vi "UDP Rx Process.vi"(10 "Parameters":variant, 11 "Process":refnum<class "Process.lvclass">) -> ()   [LabVIEW 2016, in "UDP-Custom-Device Engine.lvlib"]
uses:
  UDP-Custom-Device Engine.lvlib
  <vilib>/NI/NIVS Inline Async API/_VS Inline Async API/Process/Process.lvclass
  <vilib>/NI/NIVS Inline Async API/_VS Inline Async API/Process/Process.lvclass/Process.ctl
  <vilib>/NI Veristand/VeriStand Data/Library/Byte Buffer/Byte Buffer.lvclass/Byte Buffer.ctl
  <vilib>/NI/NIVS Inline Async API/_Data Access Engine/Access Type Classes/Write/Write.lvclass/Write.ctl
  <vilib>/NI/NIVS Inline Async API/_Data Access Engine/Data Access Engine/Methods/Write.Data.vi
  <vilib>/NI/NIVS Inline Async API/_VS Inline Async API/Process/Data Member Access/Read Data Access.vi
  <vilib>/NI/NIVS Inline Async API/_VS Inline Async API/Error Handling Process/SubVIs/Error.ConvertArray.vi
  <vilib>/NI Veristand/VeriStand Data/Library/Byte Buffer/Byte Buffer.Mapping.Read.vi
  <vilib>/NI Veristand/VeriStand Data/Library/Pointer Operations/Pointer.Read.vi
  <vilib>/NI Veristand/VeriStand Data/Library/Pointer Operations/Pointer.Read (DBL).vi
  <vilib>/NI/NIVS Inline Async API/_Data Access Engine/Access Type Classes/Write/Write.ProcessData.vi
  <vilib>/NI Veristand/VeriStand Data/Library/Type Conversion/Type Conversion.To Double.vi
  <vilib>/NI Veristand/VeriStand Data/Library/Type Conversion/Type Conversion.To Double (U16).vi
  <vilib>/NI Veristand/VeriStand Data/Library/Byte Buffer/Byte Buffer.Read.Typed Array.vi
  <vilib>/NI Veristand/VeriStand Data/Library/Memory Management/Memory Management.MoveDblBlock.Read (Double).vi
  <vilib>/NI Veristand/VeriStand Data/Library/Utilities/Utilities.Buffer.Double.vi
  <vilib>/NI Veristand/VeriStand Data/Library/Pointer Operations/Pointer.In-Place Read (DBL).vi
  <vilib>/NI Veristand/VeriStand Data/Library/Utilities/Utilities.Sizeof.Array.vi
  <vilib>/NI Veristand/VeriStand Data/Library/Byte Buffer/Byte Buffer.Read.vi
  <vilib>/NI Veristand/VeriStand Data/Library/Byte Buffer/Byte Buffer.Read (1D Boolean).vi
  <vilib>/NI Veristand/VeriStand Data/Library/Type Conversion/Type Conversion.To Double.Subset.vi
  <vilib>/NI Veristand/VeriStand Data/Library/Type Conversion/Type Conversion.To Double.Subset (1D Boolean).vi
  <vilib>/NI Veristand/VeriStand Data/Library/Byte Buffer/Byte Buffer.Read (1D SGL).vi
  <vilib>/NI Veristand/VeriStand Data/Library/Type Conversion/Type Conversion.To Double.Subset (1D SGL).vi
  <vilib>/NI Veristand/VeriStand Data/Library/Byte Buffer/Byte Buffer.Read (1D DBL).vi
  <vilib>/NI Veristand/VeriStand Data/Library/Byte Buffer/Byte Buffer.Read (1D I8).vi
  <vilib>/NI Veristand/VeriStand Data/Library/Type Conversion/Type Conversion.To Double.Subset (1D I8).vi
  <vilib>/NI Veristand/VeriStand Data/Library/Byte Buffer/Byte Buffer.Read (1D I16).vi
  <vilib>/NI Veristand/VeriStand Data/Library/Type Conversion/Type Conversion.To Double.Subset (1D I16).vi
  <vilib>/NI Veristand/VeriStand Data/Library/Byte Buffer/Byte Buffer.Read (1D I32).vi
  <vilib>/NI Veristand/VeriStand Data/Library/Type Conversion/Type Conversion.To Double.Subset (1D I32).vi
  <vilib>/NI Veristand/VeriStand Data/Library/Byte Buffer/Byte Buffer.Read (1D I64).vi
  <vilib>/NI Veristand/VeriStand Data/Library/Type Conversion/Type Conversion.To Double.Subset (1D I64).vi
  <vilib>/NI Veristand/VeriStand Data/Library/Byte Buffer/Byte Buffer.Read (1D U8).vi
  <vilib>/NI Veristand/VeriStand Data/Library/Type Conversion/Type Conversion.To Double.Subset (1D U8).vi
  <vilib>/NI Veristand/VeriStand Data/Library/Byte Buffer/Byte Buffer.Read (1D U16).vi
  <vilib>/NI Veristand/VeriStand Data/Library/Type Conversion/Type Conversion.To Double.Subset (1D U16).vi
  <vilib>/NI Veristand/VeriStand Data/Library/Byte Buffer/Byte Buffer.Read (1D U32).vi
  <vilib>/NI Veristand/VeriStand Data/Library/Type Conversion/Type Conversion.To Double.Subset (1D U32).vi
  <vilib>/NI Veristand/VeriStand Data/Library/Byte Buffer/Byte Buffer.Read (1D U64).vi
  <vilib>/NI Veristand/VeriStand Data/Library/Type Conversion/Type Conversion.To Double.Subset (1D U64).vi
  <vilib>/NI Veristand/VeriStand Data/Library/Utilities/Utilities.Sizeof.Scalar.vi
  <vilib>/NI Veristand/VeriStand Data/Library/Type Conversion/Type Conversion.To Double (1D Boolean).vi
  <vilib>/NI Veristand/VeriStand Data/Library/Type Conversion/Type Conversion.To Double (1D SGL).vi
  <vilib>/NI Veristand/VeriStand Data/Library/Type Conversion/Type Conversion.To Double (1D I8).vi
  <vilib>/NI Veristand/VeriStand Data/Library/Type Conversion/Type Conversion.To Double (1D I16).vi
  <vilib>/NI Veristand/VeriStand Data/Library/Type Conversion/Type Conversion.To Double (1D I32).vi
  <vilib>/NI Veristand/VeriStand Data/Library/Type Conversion/Type Conversion.To Double (1D I64).vi
  <vilib>/NI Veristand/VeriStand Data/Library/Type Conversion/Type Conversion.To Double (1D U8).vi
  <vilib>/NI Veristand/VeriStand Data/Library/Type Conversion/Type Conversion.To Double (1D U16).vi
  <vilib>/NI Veristand/VeriStand Data/Library/Type Conversion/Type Conversion.To Double (1D U32).vi
  <vilib>/NI Veristand/VeriStand Data/Library/Type Conversion/Type Conversion.To Double (1D U64).vi
  <vilib>/NI Veristand/VeriStand Data/Library/Byte Buffer/Byte Buffer.Set Buffer.vi
  <vilib>/NI Veristand/VeriStand Data/Library/Memory Management/Memory Management.Handle Return.vi
  <vilib>/NI/NIVS Inline Async API/_Data Access Engine/Data Access Engine/Data Access Engine.lvclass
  <vilib>/NI Veristand/VeriStand Data/Library/VeriStand Data.lvlib
panel:
  out "length":i32
  out "Rx Packet":string
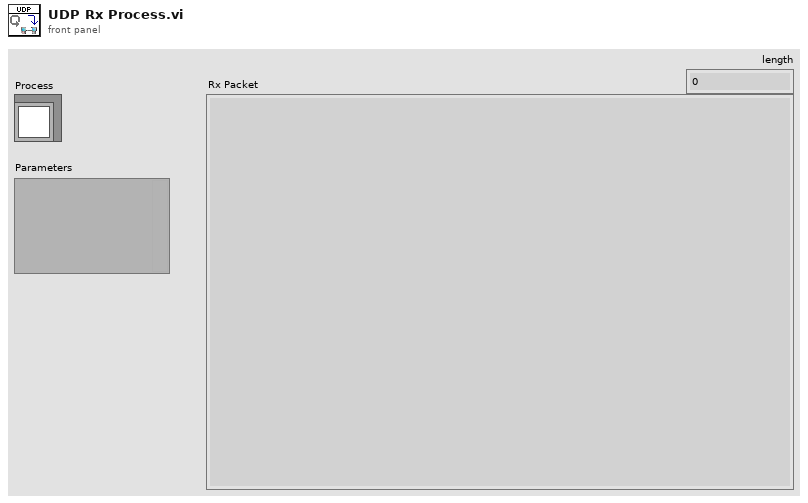
[diagram p1: front panel]
types:
  T1 = typedef "UDP-Custom-Device Engine.lvlib/Engine - Rx Loop Data.ctl" = cluster{"General Resources":T2, "Header Details":T4, "Data Conversion":T5, "Runtime Resources":T7, "New Data Support":T8, "Channel Resources":T10, "Debug Resources":T12}
  T2 = typedef "UDP-Custom-Device Engine.lvlib/Engine - General Resources.ctl" = cluster{"Packet Name":string, "Packet ID":i32, "Local IP Address":string, "Local Port":i32, "Multicast":bool, "Multicast IP Address":u32, "Header Info":bool[], "Byte Order":enum16{"big-endian, network order", "native, host order", "little-endian"}, "Channel Data Types":T3[], "Duplex Packets":refnum<data-value>}
  T3 = typedef "VeriStand Data.lvlib/Typedefs.Data Types.ctl" = enum16{"Boolean", "Single", "Double", "I8", "I16", "I32", "I64", "U8", "U16", "U32", "U64"}
  T4 = typedef "UDP-Custom-Device Shared.lvlib/Shared - Header Details.ctl" = cluster{"Packet Size":u16, "Protocol Revision":u8, "System Definition Version":u64, "Source Node Name":string, "Packet ID":u32, "Number of Channels":u32, "Static Header Size":u16, "Total Header Size":u16}
  T5 = typedef "UDP-Custom-Device Engine.lvlib/Engine - Data Conversion Config.ctl" = cluster{"Byte Buffer":refnum<class "Byte Buffer.lvclass">, "Data Pointers":u64[], "Channel Count":i32, "Mappings":T6[], "Static Header Payload":string, "Packet Count":dbl, "Packet Size":i32}
  T6 = typedef "VeriStand Data.lvlib/Byte Buffer.lvclass/Byte Buffer.Mapping.ctl" = cluster{"pointer":u64, "count":i32, "buffer offset":i32, "data type":T3}
  T7 = typedef "UDP-Custom-Device Engine.lvlib/Engine - Rx Runtime Resources.ctl" = cluster{"Connection ID":refnum<k16>, "Timeout":i32}
  T8 = typedef "UDP-Custom-Device Engine.lvlib/Engine - Rx New Data Options Support.ctl" = cluster{"New Data Option":T9, "Packet Count":dbl}
  T9 = typedef "UDP-Custom-Device Shared.lvlib/Shared - New Data Options.ctl" = enum16{"Timeout Reset", "Counter"}
  T10 = typedef "UDP-Custom-Device Engine.lvlib/Engine - Rx Channel Refs.ctl" = cluster{"Receive Channels":T11, "New Data":T11, "Port":T11}
  T11 = typedef "Data Access Engine.lvlib/Data Access Engine.lvclass/Write.DVR.ctl" = refnum<data-value>
  T12 = typedef "UDP-Custom-Device Engine.lvlib/Engine - Debug Resources.ctl" = cluster{"Debug Mode":bool, "Debug Log File":refnum<file>, "Packet Name":string}
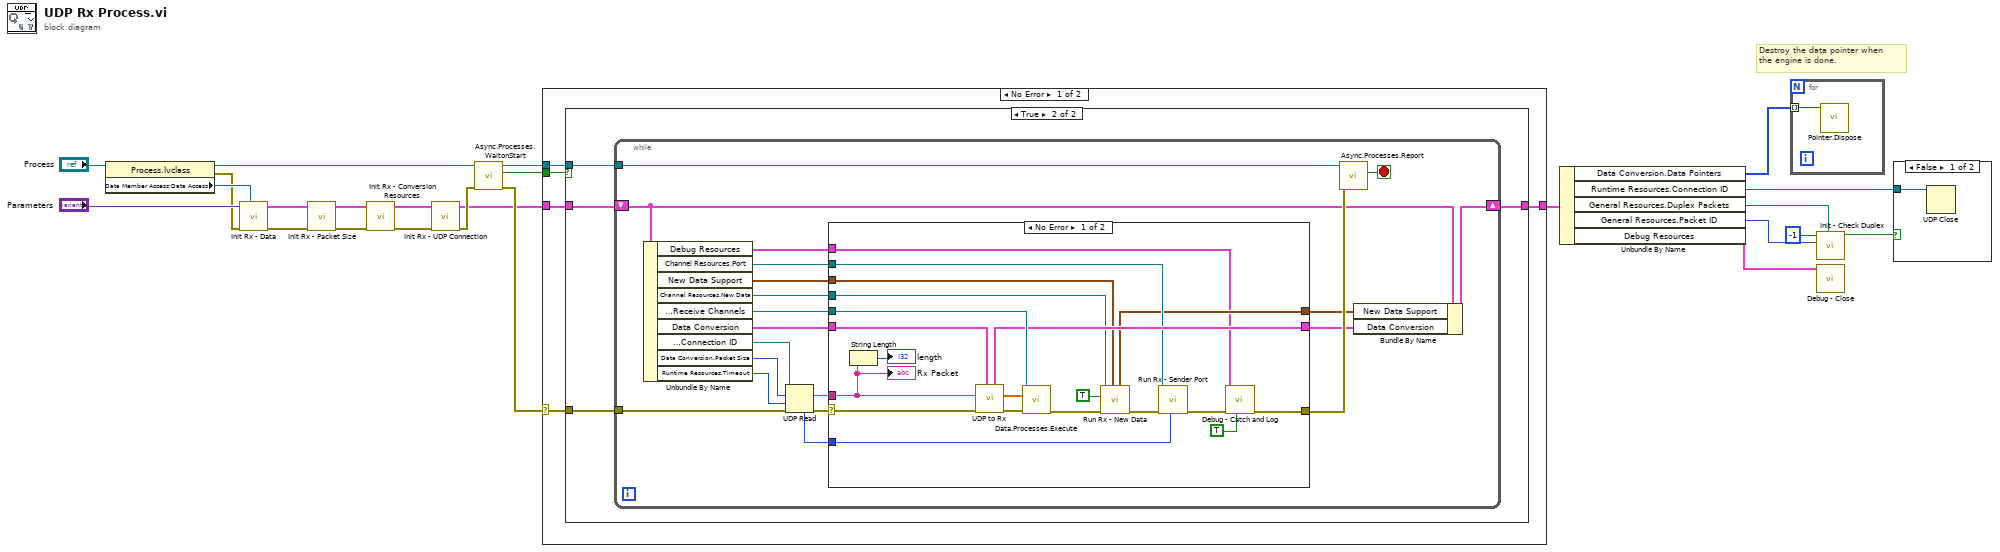
[diagram p0: block diagram]
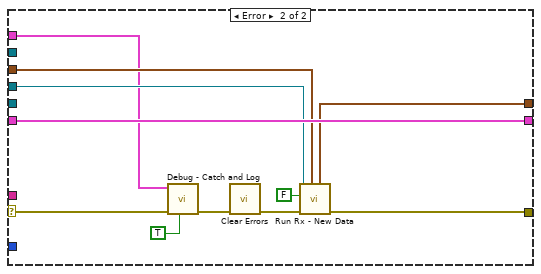
[diagram p4: hidden frame]
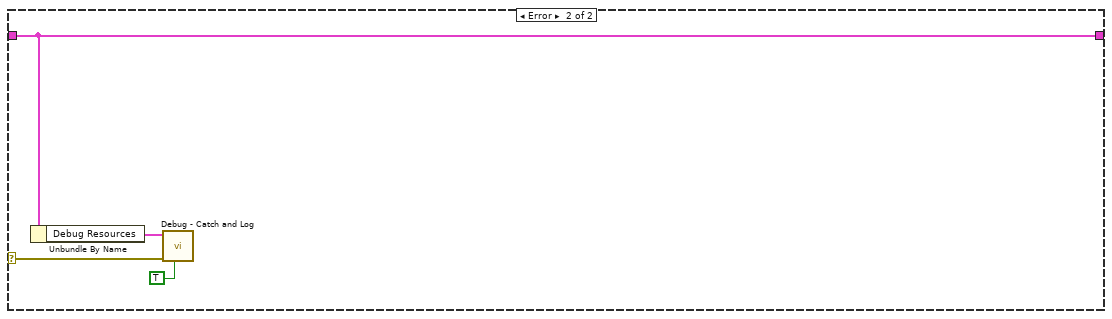
[diagram p5: hidden frame]
diagram:
  # "Destroy the data pointer when\nthe engine is done."
  n1 = property class="Process.lvclass"(reference="Process") -> (reference out=w24:refnum<class "Process.lvclass">, error out=w20:errorcluster, "Data Member Access:Data Access"=w21:refnum<class "Data Access Engine.lvclass">)  [unwired: 1 in]
  n2 = call "Init Rx - Data.vi"("Data Access in"=w21, "error in (no error)"=w20, "Parameters"="Parameters") -> ("error out"=w10:errorcluster, "Rx Loop Data"=w12:T1)  [unwired: 6 in, 1 out]
  n3 = call "Init Rx - Packet Size.vi"("error in (no error)"=w10, "Rx Loop Data"=w12) -> ("error out"=w9:errorcluster, "Rx Loop Data out"=w11:T1)  [unwired: 8 in]
  n4 = call "Init Rx - Conversion Resources.vi"("error in (no error)"=w9, "Rx Loop Data"=w11) -> ("error out"=w13:errorcluster, "Rx Loop Data out"=w14:T1)  [unwired: 8 in]
  n5 = call "Init Rx - UDP Connection.vi"("error in (no error)"=w13, "Rx Loop Data in"=w14) -> ("error out"=w16:errorcluster, "Rx Loop Data out"=w6:T1)  [unwired: 8 in]
  n6 = call <vilib>:"Async.Processes.WaitonStart.vi"("error in (no error)"=w16, "Process"=w24) -> ("error out"=w19:errorcluster, "Execute"=w17:bool, "Process out"=w18:refnum<class "Process.lvclass">)  [unwired: 7 in]
  n7 = case shown="No Error" w19 {
    selector: w19 -> [w27 w87]
    tunnel: w17 -> [w29 _]
    tunnel: w18 -> [w28 _]
    tunnel: w6 -> [w26 w86]
    tunnel: [w25 w86] -> w15
    frame No Error {
      n8 = case shown="True" w29 {
        tunnel: w27 -> [_ w33]
        tunnel: w28 -> [_ w34]
        tunnel: w26 -> [w30 w32]
        tunnel: [w30 w31] -> w25
        frame False {
        }
        frame True {
          n9 = while {
            tunnel: w33 -> [w51]
            tunnel: w34 -> [w54]
            shift-right: [w49] -> w31
            shift-left: w32 -> [w50]
            stop <- w53 stop-if-true
            n10 = Unbundle By Name(w50) -> ("Debug Resources"=w35:T12, "Channel Resources.Port"=w39:T11, "New Data Support"=w36:T8, "Channel Resources.New Data"=w43:T11, "Channel Resources.Receive Channels"=w47:T11, "Data Conversion"=w46:T5, "Runtime Resources.Connection ID"=w48:refnum<k16>, "Data Conversion.Packet Size"=w41:i32, "Runtime Resources.Timeout"=w40:i32)
            n11 = UDP Read(connection ID=w48, max size (548)=w41, timeout ms (25000)=w40, 8:w51) -> (data out=w44:string, error out=w42:errorcluster, 4:w38:u16)  [unwired: 2 out]
            n12 = case shown="No Error" w42 {
              selector: w42 -> [w66 w77]
              tunnel: [w57 w82] -> w52
              tunnel: w47 -> [w74 _]
              tunnel: w44 -> [w64 _]
              tunnel: w46 -> [w73 w85]
              tunnel: [w72 w85] -> w45
              tunnel: w43 -> [w69 w83]
              tunnel: w39 -> [w63 _]
              tunnel: w38 -> [w61 _]
              tunnel: [w60 w81] -> w37
              tunnel: w36 -> [w55 w80]
              tunnel: w35 -> [w56 w78]
              frame No Error {
                n13 = String Length(string=w64) -> (length=→"length":i32)
                n14 = call "UDP to Rx.vi"("Data Conversion"=w73, "error in (no error)"=w66, "Rx String"=w64) -> ("error out"=w71:errorcluster, "Rx Array"=w70:dbl[], "Data Conversion out"=w72:T5)  [unwired: 6 in]
                n15 = call-poly <vilib>:"Data.Processes.Execute.vi"("error in (no error)"=w71, "Values"=w70, "Ref"=w74) -> ("error out"=w68:errorcluster)  [unwired: 8 in]
                n16 = call "Run Rx - New Data.vi"("New Data Support in"=w55, "error in (no error)"=w68, "New Data"=TRUE, "New Data Ref"=w69) -> ("error out"=w62:errorcluster, "New Data Support out"=w60:T8)  [unwired: 6 in]
                n17 = call "Run Rx - Sender Port.vi"("Port"=w61, "error in (no error)"=w62, "Port Ref"=w63) -> ("error out"=w58:errorcluster)  [unwired: 8 in]
                n18 = call "Debug - Catch and Log.vi"("Clear Error?"=TRUE, "error in (no error)"=w58, "Debug Resources"=w56) -> ("error out"=w57:errorcluster)  [unwired: 8 in]
                "Rx Packet" <- w64
              }
              frame Error {
                n19 = call "Debug - Catch and Log.vi"("Clear Error?"=TRUE, "error in (no error)"=w77, "Debug Resources"=w78) -> ("error out"=w76:errorcluster)  [unwired: 8 in]
                n20 = call <vilib>:"Clear Errors.vi"("error in (no error)"=w76) -> ("error out"=w75:errorcluster)  [unwired: 5 in, 1 out]
                n21 = call "Run Rx - New Data.vi"("New Data Support in"=w80, "error in (no error)"=w75, "New Data"=FALSE, "New Data Ref"=w83) -> ("error out"=w82:errorcluster, "New Data Support out"=w81:T8)  [unwired: 6 in]
              }
            }
            n22 = call <vilib>:"Async.Processes.Report.vi"("Error"=w52, "Process in"=w54) -> ("Stop"=w53:bool)  [unwired: 8 in, 1 out]
            n23 = Bundle By Name(cluster=w50, "New Data Support"=w37, "Data Conversion"=w45) -> (w49:T1)
          }
        }
      }
    }
    frame Error {
      n24 = Unbundle By Name(w86) -> ("Debug Resources"=w88:T12)
      n25 = call "Debug - Catch and Log.vi"("Clear Error?"=TRUE, "error in (no error)"=w87, "Debug Resources"=w88) -> ()  [unwired: 8 in, 1 out]
    }
  }
  n26 = Unbundle By Name(w15) -> ("Data Conversion.Data Pointers"=w8:u64[], "Runtime Resources.Connection ID"=w7:refnum<k16>, "General Resources.Duplex Packets"=w2:refnum<data-value>, "General Resources.Packet ID"=w4:i32, "Debug Resources"=w1:T12)
  n27 = for {
    tunnel: w8 -> [w90] mode=indexing
    n28 = call <vilib>:"Pointer.Dispose.vi"("pointer"=w90) -> ()  [unwired: 9 in, 2 out]
  }
  n29 = call "Init - Check Duplex.vi"("Duplex Packets"=w2, "Receive Packet ID"=w4, "Transmit Packet ID"=-1 ("Receive Packet ID")) -> ("Is Duplex?"=w3:bool)  [unwired: 6 in, 2 out]
  n30 = call "Debug - Close.vi"("Debug Resources"=w1) -> ()  [unwired: 10 in, 1 out]
  n31 = case shown="False" w3 {
    tunnel: w7 -> [w91 _]
    frame False {
      n32 = UDP Close(connection ID=w91) -> ()  [unwired: 1 in, 2 out]
    }
    frame True {
    }
  }
